vi "programa 2.vi"() -> ()   [LabVIEW 2011]
uses:
  control del programa 2.ctl
panel:
  out "Array":T1(array[cluster]) {"Velocidad3" scale=0.0..180.0; "Velocidad2" scale=0.0..180.0; "Velocidad1" scale=0.0..180.0}
  # "Se tiene que ingresar las 3 velocidades de cada elemento del arreglo\nluego se debara de obtener el promedio de cada uno de los elmentos del arreglo.\n\nIniciar arreglo, rellenar arreglo, obtener promedio, finalizar."
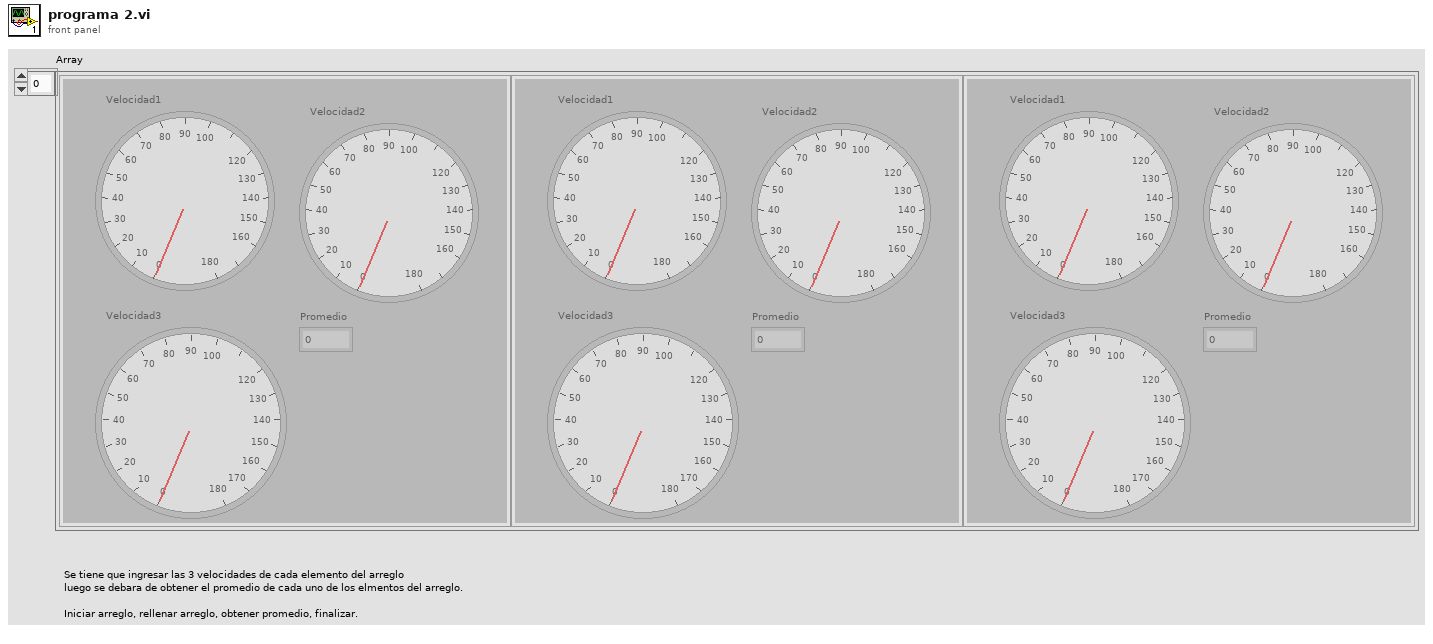
[diagram p1: front panel]
types:
  T1 = cluster{"Velocidad1":i32, "Velocidad2":i32, "Velocidad3":i32, "Promedio":dbl}[]
  T2 = typedef "control del programa 2.ctl" = enum16{"Iniciar arreglo", "Rellenar arreglo", "Obtener promedio", "Finalizar"}
  T3 = cluster{"Velocidad1":i32, "Velocidad2":i32, "Velocidad3":i32, "Promedio":dbl}
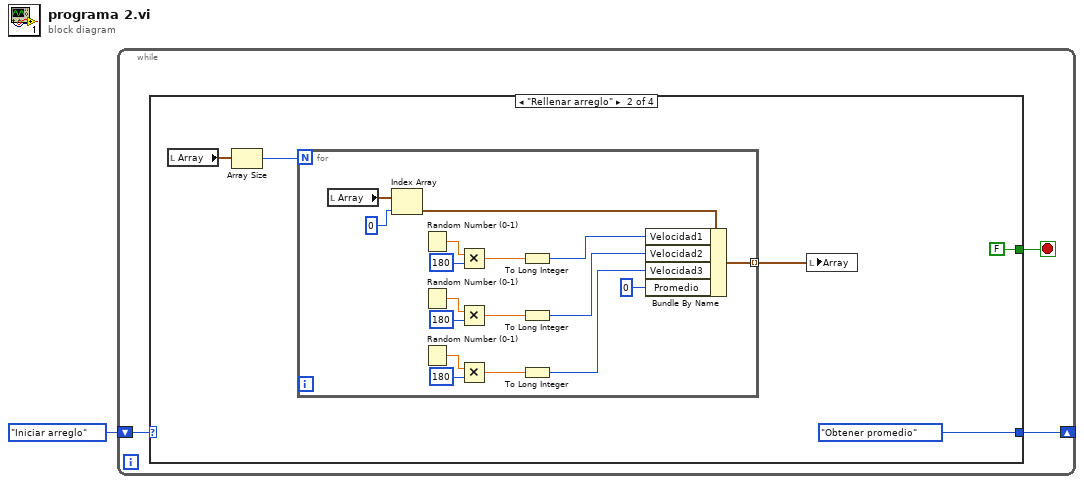
[diagram p0: block diagram]
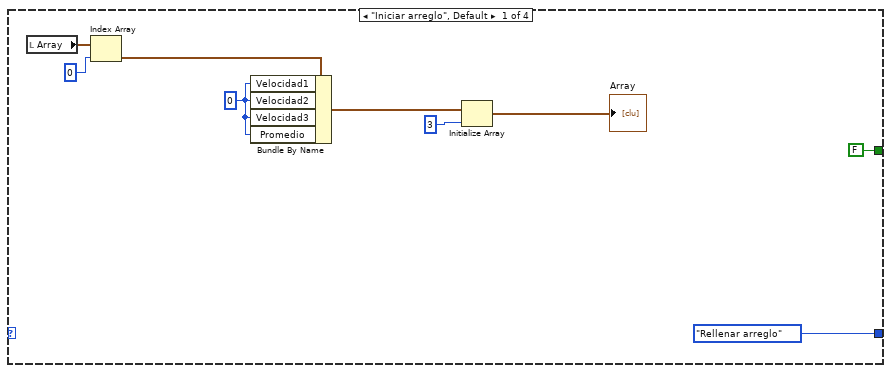
[diagram p2: hidden frame]
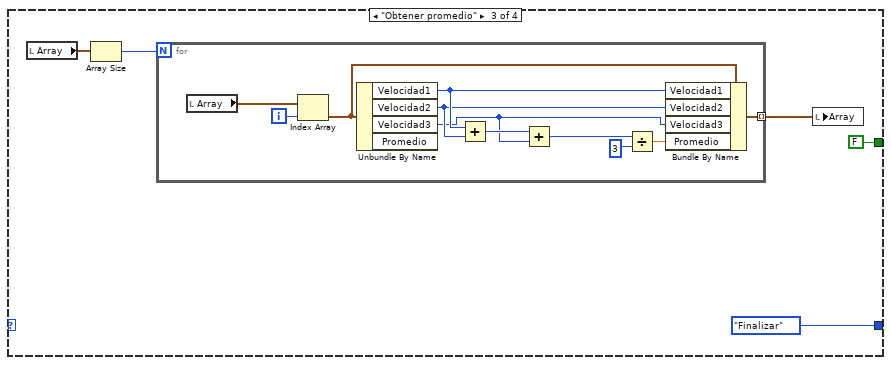
[diagram p3: hidden frame]
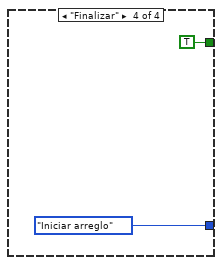
[diagram p4: hidden frame]
diagram:
  n1 = while {
    shift-right: [w3] -> _
    shift-left: control_del_programa_2."Iniciar arreglo" -> [w4]
    stop <- w2 stop-if-true
    n2 = case shown="\"Rellenar arreglo\"" w4 {
      tunnel: [control_del_programa_2."Rellenar arreglo" control_del_programa_2."Obtener promedio" control_del_programa_2."Finalizar" control_del_programa_2."Iniciar arreglo"] -> w3
      tunnel: [FALSE FALSE FALSE TRUE] -> w2
      frame "Iniciar arreglo", Default {
        w10 = 0
        n3 = local read "Array"() -> (w13:T1)
        n4 = Index Array "Index Array"(array=w13, index=0) -> (element=w11:T3)
        n5 = Bundle By Name "Bundle By Name"(cluster=w11, "Velocidad1"=w10, "Velocidad2"=w10, "Velocidad3"=w10, "Promedio"=w10) -> (w8:T3)
        n6 = Initialize Array "Initialize Array"(w8, 3) -> (→"Array":T1)
      }
      frame "Rellenar arreglo" {
        n7 = local read "Array"() -> (w17:T1)
        n8 = Array Size(array=w17) -> (size(s)=w18:i32)
        n9 = for {
          N: w18 -> [_]
          tunnel: [w19] -> w16 mode=indexing
          n10 = local read "Array"() -> (w35:T1)
          n11 = Index Array "Index Array"(array=w35, index=0) -> (element=w33:T3)
          n12 = Random Number (0-1)() -> (number: 0 to 1=w31:dbl)
          n13 = Random Number (0-1)() -> (number: 0 to 1=w28:dbl)
          n14 = Random Number (0-1)() -> (number: 0 to 1=w25:dbl)
          n15 = Multiply(x=w31, y=180) -> (x*y=w32:dbl)
          n16 = Multiply(x=w28, y=180) -> (x*y=w27:dbl)
          n17 = Multiply(x=w25, y=180) -> (x*y=w26:dbl)
          n18 = To Long Integer(number=w32) -> (32bit integer=w23:i32)
          n19 = To Long Integer(number=w27) -> (32bit integer=w22:i32)
          n20 = To Long Integer(number=w26) -> (32bit integer=w21:i32)
          n21 = Bundle By Name "Bundle By Name"(cluster=w33, "Velocidad1"=w23, "Velocidad2"=w22, "Velocidad3"=w21, "Promedio"=0) -> (w19:T3)
        }
        n22 = local write "Array"(w16) -> ()
      }
      frame "Obtener promedio" {
        n23 = local read "Array"() -> (w39:T1)
        n24 = Array Size(array=w39) -> (size(s)=w40:i32)
        n25 = for {
          N: w40 -> [_]
          tunnel: [w45] -> w37 mode=indexing
          i -> [w47]
          n26 = local read "Array"() -> (w51:T1)
          n27 = Index Array(array=w51, index=w47) -> (element=w48:T3)
          n28 = Unbundle By Name(w48) -> ("Velocidad1"=w44:i32, "Velocidad2"=w43:i32, "Velocidad3"=w42:i32)  [unwired: 1 out]
          n29 = Add(x=w44, y=w43) -> (x+y=w50:i32)
          n30 = Add(x=w50, y=w42) -> (x+y=w49:i32)
          n31 = Divide(x=w49, y=3) -> (x/y=w46:dbl)
          n32 = Bundle By Name(cluster=w48, "Velocidad1"=w44, "Velocidad2"=w43, "Velocidad3"=w42, "Promedio"=w46) -> (w45:T3)
        }
        n33 = local write "Array"(w37) -> ()
      }
      frame "Finalizar" {
      }
    }
  }
